vi "Skip Failure Check.vi"(10 "Test Name Prefix":string, 11 "Test Name Input":string) -> (3 "Skip Failure Check?":bool)   [LabVIEW 2018, in "STDF File Parser.lvclass"]
uses:
  STDF File Parser.lvclass
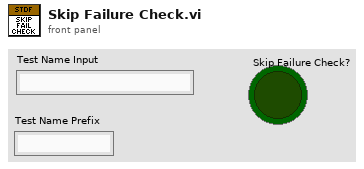
[diagram p1: front panel]
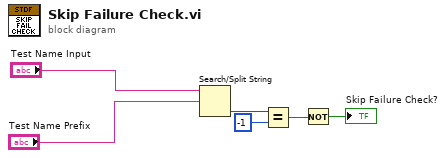
[diagram p0: block diagram]
diagram:
  n1 = Search/Split String(string="Test Name Input", search string/char (-)="Test Name Prefix") -> (offset of match=w4:i32)  [unwired: 1 in, 2 out]
  n2 = Equal?(x=w4, y=-1) -> (x = y?=w2:bool)
  n3 = Not(x=w2) -> (.not. x?=→"Skip Failure Check?":bool)
